vi "Configure IQ Adjustment.vi"(0 "VISA resource name":refnum<visa-resource-name>, 1 "I Offset (0 percent)":dbl, 2 "Enable I/Q Adjustment (F:Disable)":bool, 5 "Q Offset (0 percent)":dbl, 7 "Gain (0 dB)":dbl, 9 "Quadrature Skew (0 deg)":dbl, 11 "error in (no error)":errorcluster, 12 "I/Q Skew (0 s)":dbl, 13 "I/Q Timing Skew Path (0: RF)":u16(ring) items=["RF", "Baseband"], 14 "I/Q Delay (0 s)":dbl) -> (4 "VISA resource name out":refnum<visa-resource-name>, 15 "error out":errorcluster)   [LabVIEW 2014, in "Agilent PSG MXG Series.lvlib"]
doc: "Configures I/Q adjustments.\n\n<B>Notes:</B>\n(1) This VI is valid only in E8267C, E8267D, N5162A, N5182A, N5172B, N5182B.\n\n(2) For E8267C, this VI is valid only when the instrument installs <B>Option 002</B> (Internal baseband generator) or <B>Option 602</B> (Digital bus baseband generator)."
uses:
  Agilent PSG MXG Series.lvlib
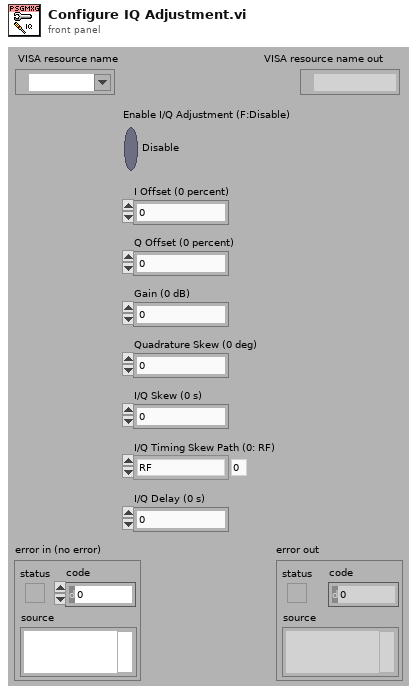
[diagram p1: front panel]
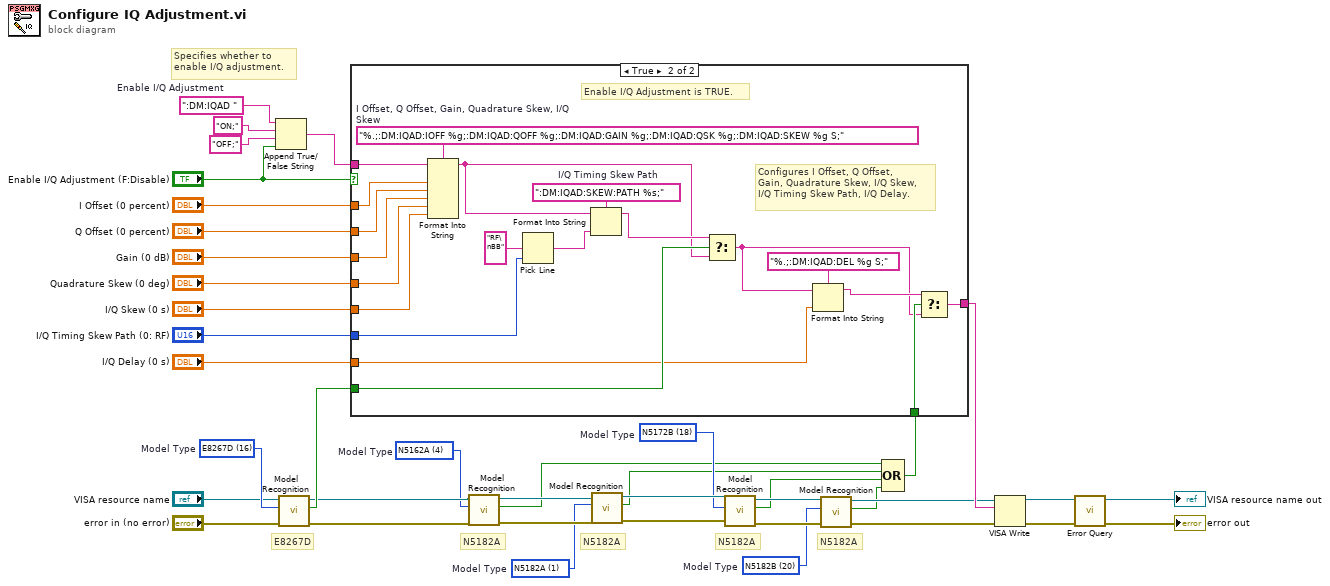
[diagram p0: block diagram]
diagram:
  w6 = u16 20 items=["N5181A"=0, "N5182A"=1, "N5183A"=2, "N5161A"=3, "N5162A"=4, "E8241A"=5, "E8244A"=6, "E8251A"=7, "E8254A"=8, "E8247C"=10, "E8257C"=11, "E8267C"=12, "E8257D"=15, "E8267D"=16, "N5171B"=17, "N5172B"=18, "N5181B"=19, "N5182B"=20]  # Model Type
  w7 = u16 18 items=["N5181A"=0, "N5182A"=1, "N5183A"=2, "N5161A"=3, "N5162A"=4, "E8241A"=5, "E8244A"=6, "E8251A"=7, "E8254A"=8, "E8247C"=10, "E8257C"=11, "E8267C"=12, "E8257D"=15, "E8267D"=16, "N5171B"=17, "N5172B"=18, "N5181B"=19, "N5182B"=20]  # Model Type
  w8 = u16 4 items=["N5181A"=0, "N5182A"=1, "N5183A"=2, "N5161A"=3, "N5162A"=4, "E8241A"=5, "E8244A"=6, "E8251A"=7, "E8254A"=8, "E8247C"=10, "E8257C"=11, "E8267C"=12, "E8257D"=15, "E8267D"=16, "N5171B"=17, "N5172B"=18, "N5181B"=19, "N5182B"=20]  # Model Type
  w9 = u16 1 items=["N5181A"=0, "N5182A"=1, "N5183A"=2, "N5161A"=3, "N5162A"=4, "E8241A"=5, "E8244A"=6, "E8251A"=7, "E8254A"=8, "E8247C"=10, "E8257C"=11, "E8267C"=12, "E8257D"=15, "E8267D"=16, "N5171B"=17, "N5172B"=18, "N5181B"=19, "N5182B"=20]  # Model Type
  w24 = u16 16 items=["N5181A"=0, "N5182A"=1, "E8241A"=5, "E8244A"=6, "E8251A"=7, "E8254A"=8, "E8247C"=10, "E8257C"=11, "E8267C"=12, "E8257D"=15, "E8267D"=16]  # Model Type
  w39 = ":DM:IQAD "  # Enable I/Q Adjustment
  # "N5182A"
  # "N5182A"
  # "N5182A"
  # "Specifies whether to\nenable I/Q adjustment."
  # "E8267D"
  # "N5182A"
  n1 = Append True/False String(1:"Enable I/Q Adjustment (F:Disable)", 2:"OFF;" ("false string"), 3:"ON;" ("true string"), 4:w39) -> (0:w35:string)
  n2 = call "Model Recognition.vi"("error in (no error)"="error in (no error)", "Model Type (0: N5181A)"=w24, "VISA resource name"="VISA resource name") -> ("error out"=w15:errorcluster, "Is Model Correct"=w23:bool, "VISA resource name out"=w10:refnum<visa-resource-name>)  [unwired: 6 out]
  n3 = call "Model Recognition.vi"("error in (no error)"=w15, "Model Type (0: N5181A)"=w8, "VISA resource name"=w10) -> ("error out"=w14:errorcluster, "Is Model Correct"=w2:bool, "VISA resource name out"=w11:refnum<visa-resource-name>)  [unwired: 6 out]
  n4 = call "Model Recognition.vi"("error in (no error)"=w14, "Model Type (0: N5181A)"=w9, "VISA resource name"=w11) -> ("error out"=w13:errorcluster, "Is Model Correct"=w3:bool, "VISA resource name out"=w12:refnum<visa-resource-name>)  [unwired: 6 out]
  n5 = call "Model Recognition.vi"("error in (no error)"=w13, "Model Type (0: N5181A)"=w7, "VISA resource name"=w12) -> ("error out"=w22:errorcluster, "Is Model Correct"=w4:bool, "VISA resource name out"=w17:refnum<visa-resource-name>)  [unwired: 6 out]
  n6 = call "Model Recognition.vi"("Model Type (0: N5181A)"=w6, "VISA resource name"=w17) -> ("Is Model Correct"=w5:bool, "VISA resource name out"=w16:refnum<visa-resource-name>)  [unwired: 1 in, 7 out]
  n7 = Compound Arithmetic op=OR(w2, w3, w4, w5) -> (w1:bool)
  n8 = case shown="True" "Enable I/Q Adjustment (F:Disable)" {
    tunnel: w35 -> [w40 w59]
    tunnel: "I Offset (0 percent)" -> [_ w58]
    tunnel: "Q Offset (0 percent)" -> [_ w57]
    tunnel: "Gain (0 dB)" -> [_ w56]
    tunnel: "Quadrature Skew (0 deg)" -> [_ w55]
    tunnel: "I/Q Skew (0 s)" -> [_ w54]
    tunnel: "I/Q Timing Skew Path (0: RF)" -> [_ w52]
    tunnel: w23 -> [_ w49]
    tunnel: "I/Q Delay (0 s)" -> [_ w45]
    tunnel: w1 -> [_ w44]
    tunnel: [w40 w41] -> w27
    frame False {
      # "Enable I/Q Adjustment is FALSE."
    }
    frame True {
      w51 = ":DM:IQAD:SKEW:PATH %s;"  # I/Q Timing Skew Path
      w60 = "%.;:DM:IQAD:IOFF %g;:DM:IQAD:QOFF %g;:DM:IQAD:GAIN %g;:DM:IQAD:QSK %g;:DM:IQAD:SKEW %g S;"  # I Offset, Q Offset, Gain, Quadrature Skew, I/Q Skew
      # "Configures I Offset, Q Offset,\nGain, Quadrature Skew, I/Q Skew,\nI/Q Timing Skew Path, I/Q Delay."
      # "Enable I/Q Adjustment is TRUE."
      n9 = Format Into String(format string=w60, initial string=w59, w58, w57, w56, w55, w54) -> (resulting string=w47:string)  [unwired: 1 in, 1 out]
      n10 = Pick Line(multi-line string="RF\nBB", line index=w52) -> (output string=w50:string)  [unwired: 1 out]
      n11 = Format Into String(format string=w51, initial string=w47, w50) -> (resulting string=w48:string)  [unwired: 1 in, 1 out]
      n12 = Select(t=w48, s=w49, f=w47) -> (s? t:f=w42:string)
      n13 = Format Into String(format string="%.;:DM:IQAD:DEL %g S;", initial string=w42, w45) -> (resulting string=w43:string)  [unwired: 1 in, 1 out]
      n14 = Select(t=w43, s=w44, f=w42) -> (s? t:f=w41:string)
    }
  }
  n15 = VISA Write(VISA resource name=w16, write buffer=w27, error in (no error)=w22) -> (VISA resource name out=w26:refnum<visa-resource-name>, error out=w25:errorcluster)  [unwired: 1 out]
  n16 = call "Error Query.vi"("error in (no error)"=w25, "VISA resource name"=w26) -> ("error out"=→"error out":errorcluster, "VISA resource name out"=→"VISA resource name out":refnum<visa-resource-name>)  [unwired: 8 out]
